vi "Get Custom Device.vi"(8 "error in":errorcluster, 11 "custom device ref in":T1 format="%.0x") -> (0 "error out":errorcluster, 1 "Item Refs":T1[](array[typedef]) format="%.0x", 2 "First Item Ref":T1 format="%.0x", 3 "custom device ref out":T1 format="%.0x", 4 "Found":bool)   [LabVIEW 2020, in "AIM ARINC 664 Scripting.lvlib"]
doc: "This VI allows you to obtain all of the AIM ARINC 664 custom devices available in the system definition. It also returns the first one available, in case you only have one Custom Device."
uses:
  AIM ARINC 664 Scripting.lvlib
  <vilib>/NI VeriStand/Custom Device Tools/Custom Device Utility Library/Custom Device Utility Library.lvlib
  Constants.vi
  <vilib>/NI VeriStand/Custom Device Tools/Custom Device Utility Library/NI VeriStand - Search for All Items by GUID.vi
  <vilib>/NI VeriStand/Custom Device API/Custom Device Item Ref.ctl
  <vilib>/NI VeriStand/Custom Device API/Custom Device API.lvlib
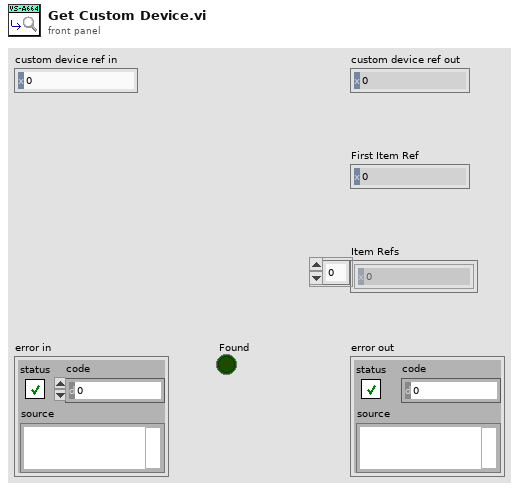
[diagram p1: front panel]
types:
  T1 = typedef "Custom Device API.lvlib/Custom Device Item Ref.ctl" = u64
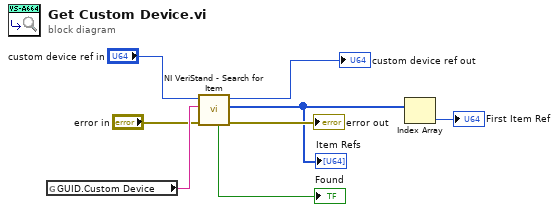
[diagram p0: block diagram]
diagram:
  n1 = global read "Constants.vi" "GUID.Custom Device"() -> (w8:string)
  n2 = call-poly <vilib>:"NI VeriStand - Search for Item.vi"("error in"="error in", "Item GUID"=w8, "Section Ref in"="custom device ref in") -> ("error out"=→"error out":errorcluster, "Item Refs"=w2:T1[], "Section Ref out"=→"custom device ref out":T1, "Found"=→"Found":bool)  [unwired: 5 in]
  "Item Refs" <- w2
  n3 = Index Array(array=w2) -> (element=→"First Item Ref":T1)  [unwired: 1 in]
